vi "MGI Debug Window Message.vi"(10 "error in (no error)":errorcluster, 11 "Mesage (Null:Closes Window)":string="\u0000") -> (2 "error out":errorcluster)   [LabVIEW 2016]
doc: "Add the specified text to a line of a special LabVIEW debug window that will show the first time a message is added. This is a useful tool for debugging.\n\nThe window may be programatically closed by calling this VI with the Null character string (\"\\0\")\n\nAuthored by Shawn Walpole\nsupport@mooregoodideas.com\nwww.mooregoodideas.com\n\nCopyright (c) 2010, Moore Good Ideas, Inc.\n\nAll rights reserved.\n\nRedistribution and use in source and binary forms, with or without modification, are permitted provided that the following conditions are met:\n\n * Redistributions of source code must retain the above copyright notice, this list of conditions and the following disclaimer.\n * Redistributions in binary form must reproduce the above copyright notice, this list of conditions and the following disclaimer in the documentation and/or other materials provided with the distribution.\n * Neither the name of Moore Good Ideas, Inc. nor the names of its contributors may be used to endorse or promote products derived from this software without specific prior written permission.\n\nTHIS SOFTWARE IS PROVIDED BY THE COPYRIGHT HOLDERS AND CONTRIBUTORS \"AS IS\" AND ANY EXPRESS OR IMPLIED WARRANTIES, INCLUDING, BUT NOT LIMITED TO, THE IMPLIED WARRANTIES OF MERCHANTABILITY AND FITNESS FOR A PARTICULAR PURPOSE ARE DISCLAIMED. IN NO EVENT SHALL THE COPYRIGHT OWNER OR CONTRIBUTORS BE LIABLE FOR ANY DIRECT, INDIRECT, INCIDENTAL, SPECIAL, EXEMPLARY, OR CONSEQUENTIAL DAMAGES (INCLUDING, BUT NOT LIMITED TO, PROCUREMENT OF SUBSTITUTE GOODS OR SERVICES; LOSS OF USE, DATA, OR PROFITS; OR BUSINESS INTERRUPTION) HOWEVER CAUSED AND ON ANY THEORY OF LIABILITY, WHETHER IN CONTRACT, STRICT LIABILITY, OR TORT (INCLUDING NEGLIGENCE OR OTHERWISE) ARISING IN ANY WAY OUT OF THE USE OF THIS SOFTWARE, EVEN IF ADVISED OF THE POSSIBILITY OF SUCH DAMAGE."
uses:
  LabVIEW.exe
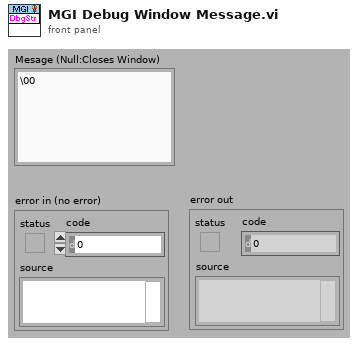
[diagram p1: front panel]
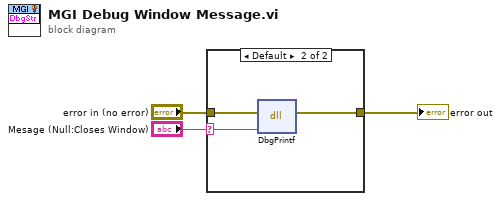
[diagram p0: block diagram]
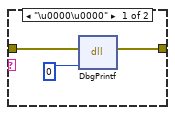
[diagram p2: hidden frame]
diagram:
  n1 = case shown="Default" "Mesage (Null:Closes Window)" {
    selector: "Mesage (Null:Closes Window)" -> [_ w7]
    tunnel: "error in (no error)" -> [w5 w9]
    tunnel: [w4 w8] -> w1
    frame "\u0000\u0000" {
      n2 = dll-call lib="LabVIEW.exe" fn="DbgPrintf"(error in=w5, "arg1"=0) -> (error out=w4:errorcluster)  [unwired: 4 in, 1 out]
    }
    frame Default {
      n3 = dll-call lib="LabVIEW.exe" fn="DbgPrintf"(error in=w9, "arg1"=w7) -> (error out=w8:errorcluster)  [unwired: 4 in, 1 out]
    }
  }
  "error out" <- w1
